vi "Send Query Arb Waveform Capabilities 64 [ARB64].vi"(7 "Message Priority (Normal)":T1=enum."Normal", 8 "error in (no error)":errorcluster, 11 "Message Enqueuer":refnum<class "Message Enqueuer.lvclass">) -> (0 "error out":errorcluster, 3 "Message Enqueuer out":refnum<class "Message Enqueuer.lvclass">)   [LabVIEW 2015, in "CS++Fgen.lvlib" / "Query Arb Waveform Capabilities 64 [ARB64] Msg.lvclass"]
doc: "Sends the <B>CS++Fgen.lvlib:Query Arb Waveform Capabilities 64 [ARB64] Msg.lvclass</B> message.\n\n<B>CS++Fgen.lvlib:CS++Fgen.lvclass:Query Arb Waveform Capabilities 64 [ARB64].vi</B> Description:\n\nThis VI returns the properties of the function generator that are related to creating arbitrary waveforms. These properties are the maximum number of waveforms, waveform quantum, minimum waveform size, and maximum waveform size.\n\nThis VI is a 64-bit version of IviFgen Query Arb Waveform Capabilities [ARB] VI.\n\nNote:\n\n(1) This VI is part of the IviFgenArbWfmSize64 [ARB64] extension group."
uses:
  Query Arb Waveform Capabilities 64 [ARB64] Msg.lvclass
  <vilib>/ActorFramework/Message Enqueuer/Message Enqueuer.lvclass
  <vilib>/ActorFramework/Message Enqueuer/Message Priority.ctl
  <vilib>/ActorFramework/Message Enqueuer/Message Enqueuer.lvclass/Message Enqueuer.ctl
  <vilib>/ActorFramework/Message Priority Queue/Priority Enqueue.vi
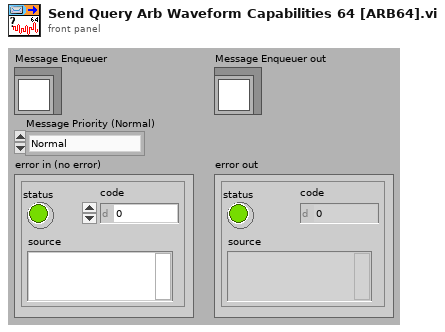
[diagram p1: front panel]
types:
  T1 = typedef "Actor Framework.lvlib/Message Enqueuer.lvclass/Message Priority.ctl" = enum16{"Low", "Normal", "High"}
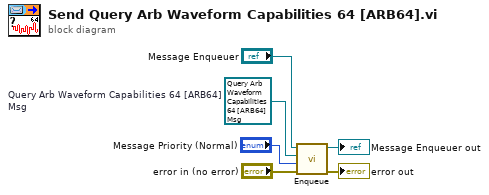
[diagram p0: block diagram]
diagram:
  w1 = refnum<class "Query Arb Waveform Capabilities 64 [ARB64] Msg.lvclass"> refnum  # Query Arb Waveform Capabilities 64 [ARB64] Msg
  n1 = call <vilib>:"Enqueue.vi"("error in (no error)"="error in (no error)", "Message Priority (Normal)"="Message Priority (Normal)", "Message"=w1, "Message Enqueuer in"="Message Enqueuer") -> ("error out"=→"error out":errorcluster, "Message Enqueuer out"=→"Message Enqueuer out":refnum<class "Message Enqueuer.lvclass">)  [unwired: 6 in]
